vi "Update Z-Cursors Positions.vi"(8 "error in":errorcluster, 9 "Length":i32, 10 "Index":i32, 11 "Series Graph in":refnum<vi>) -> (0 "error out":errorcluster)   [LabVIEW 2023, in "Graph with Analysis Controls.lvclass"]
uses:
  Graph with Analysis Controls.lvclass
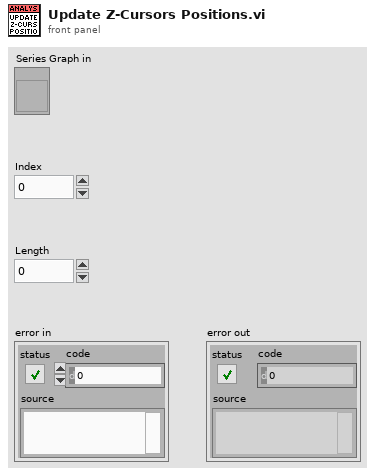
[diagram p1: front panel]
types:
  T1 = typedef "LVCursorListTypeDef.ctl" = cluster{"Name":string, "Color":u32, "Style":u8, "Point Style":u8, "Name Visible":bool, "Allow Drag":bool, "Cursor Mode":u32, "Plot":i32, "Index":i32, "Position":cluster{"X":dbl, "Y":dbl}, "X Scale":u32, "Y Scale":u32, "Watch Plots":i32[], "Watch All Plots":bool, "Plot Area":i32, "Label Offset":cluster{"X":dbl, "Y":dbl}}[]
  T2 = cluster{"Name":string, "Color":u32, "Style":u8, "Point Style":u8, "Name Visible":bool, "Allow Drag":bool, "Cursor Mode":u32, "Plot":i32, "Index":i32, "Position":cluster{"X":dbl, "Y":dbl}, "X Scale":u32, "Y Scale":u32, "Watch Plots":i32[], "Watch All Plots":bool, "Plot Area":i32, "Label Offset":cluster{"X":dbl, "Y":dbl}}
  T3 = cluster{"Name":string, "Color":u32, "Style":u8, "Point Style":u8, "Name Visible":bool, "Allow Drag":bool, "Cursor Mode":u32, "Plot":i32, "Index":i32, "Position":cluster{"X":dbl, "Y":dbl}, "X Scale":u32, "Y Scale":u32, "Watch Plots":i32[], "Watch All Plots":bool, "Plot Area":i32, "Label Offset":cluster{"X":dbl, "Y":dbl}}[]
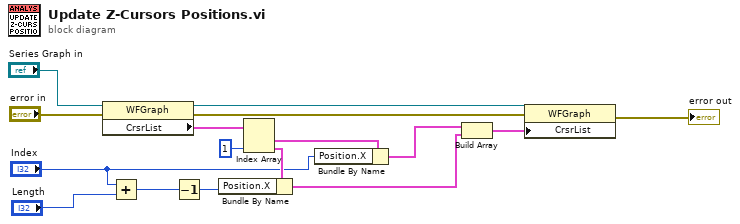
[diagram p0: block diagram]
diagram:
  n1 = property on="Property Node" class="WFGraph"(reference="Series Graph in", error in="error in") -> (reference out=w10:refnum<vi>, error out=w9:errorcluster, "CrsrList"=w11:T1)
  n2 = Add(x="Index", y="Length") -> (x+y=w2:i32)
  n3 = Decrement(x=w2) -> (x-1=w1:i32)
  n4 = Index Array(array=w11, index #2=1 ("index")) -> (element #1=w15:T2, element #2=w16:T2)  [unwired: 1 in]
  n5 = Bundle By Name(cluster=w16, "Position.X"=w1) -> (w6:T2)
  n6 = Bundle By Name(cluster=w15, "Position.X"="Index") -> (w7:T2)
  n7 = Build Array(w7, w6) -> (w8:T3)
  n8 = property on="Property Node" class="WFGraph"(reference=w10, error in=w9, "CrsrList"=w8) -> (error out=→"error out":errorcluster)  [unwired: 1 out]
